vi "LV message server.vi"() -> ()   [LabVIEW 2019, in "mmW_commands.lvlib"]
uses:
  <vilib>/addons/zeromq/socket_type.ctl
  <vilib>/Waveform/WDTOps.llb/WDT Number of Waveform Samples DBL.vi
  mmW_commands.lvlib
  <vilib>/addons/zeromq/zmq_context.lvclass
  <vilib>/addons/zeromq/zmq_socket.lvclass
  <vilib>/addons/zeromq/zeromq.lvlib
  <vilib>/measure/NI_MABase.lvlib
panel:
  out "Config":cluster{"Instrument":string, "Fs":dbl}
  out "size(s)":i32
  out "TX data":waveform(dbl)(graph)
  out "message history":string[](array[string])
  out "error out":errorcluster
  in  "Stop Button":bool
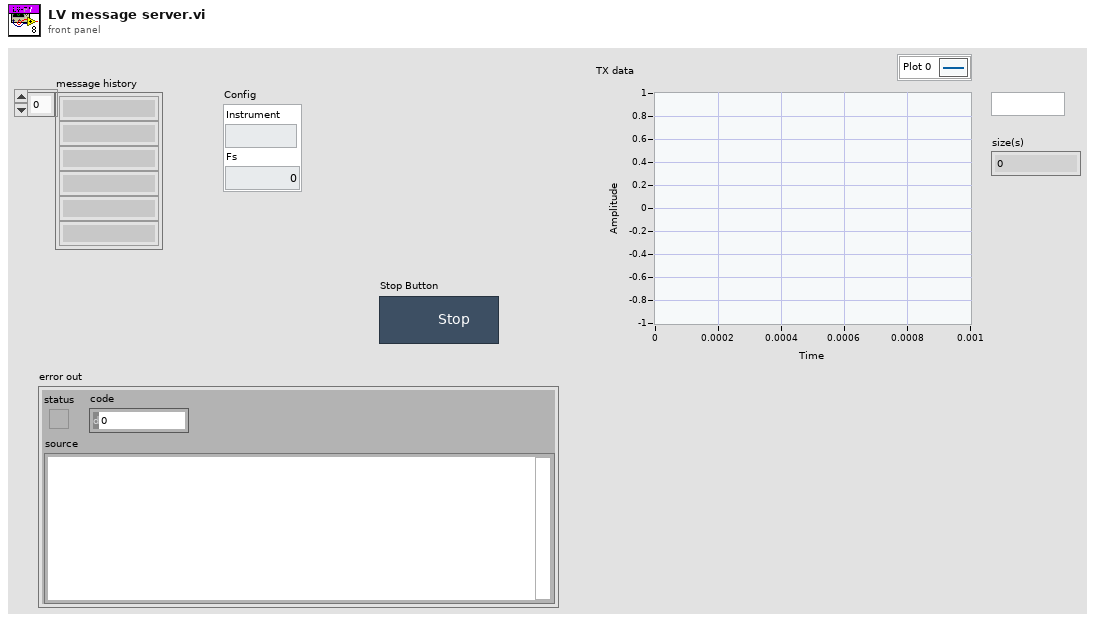
[diagram p1: front panel]
types:
  T1 = typedef "zeromq.lvlib/socket_type.ctl" = enum8{"ZMQ_PAIR", "ZMQ_PUB", "ZMQ_SUB", "ZMQ_REQ", "ZMQ_REP", "ZMQ_DEALER", "ZMQ_ROUTER", "ZMQ_PULL", "ZMQ_PUSH", "ZMQ_XPUB", "ZMQ_XSUB"}
  T2 = enum16{"big-endian, network order", "native, host order", "little-endian"}
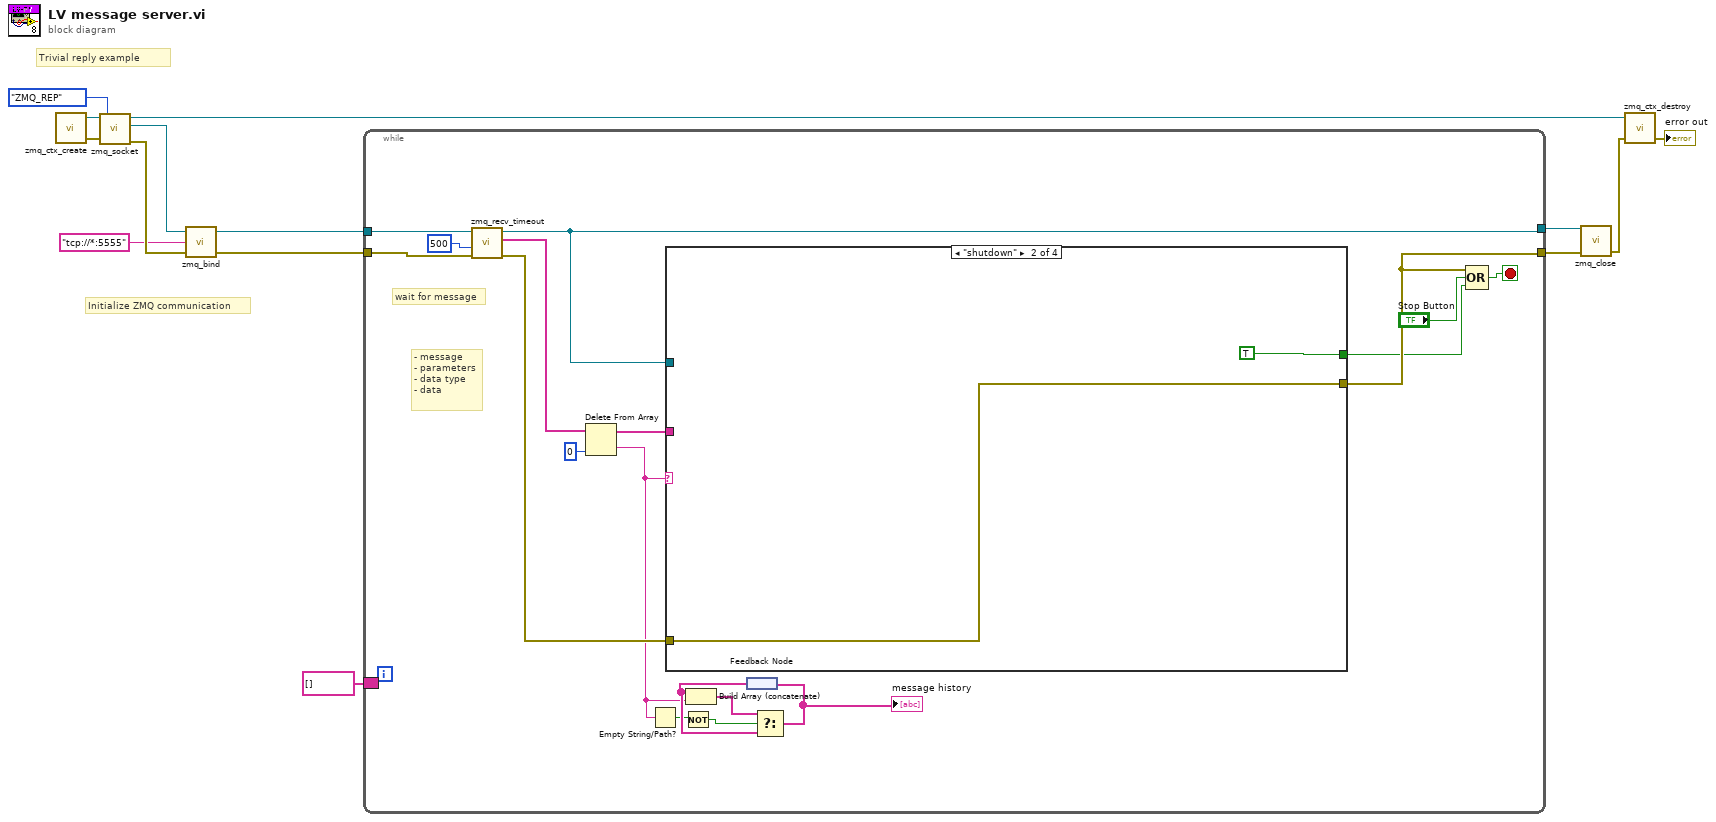
[diagram p0: block diagram]
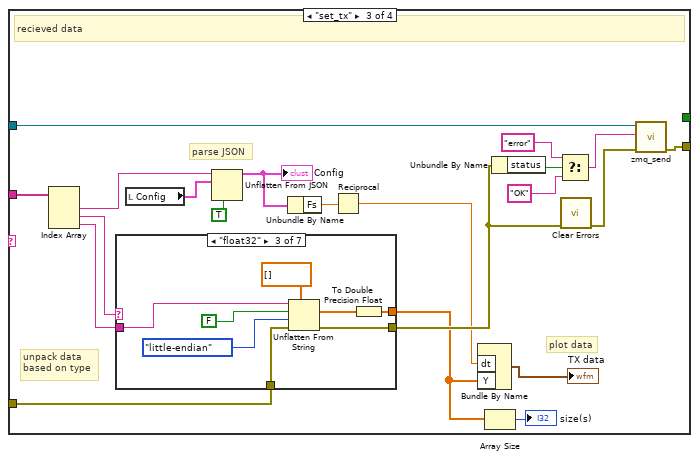
[diagram p3: hidden frame]
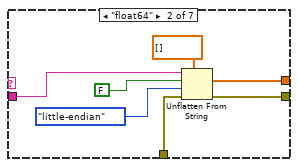
[diagram p5: hidden frame]
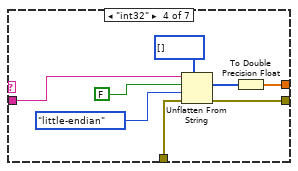
[diagram p6: hidden frame]
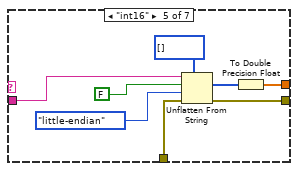
[diagram p7: hidden frame]
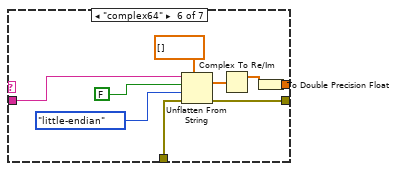
[diagram p8: hidden frame]
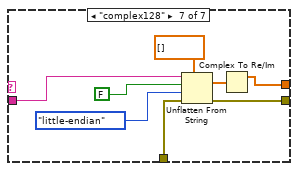
[diagram p9: hidden frame]
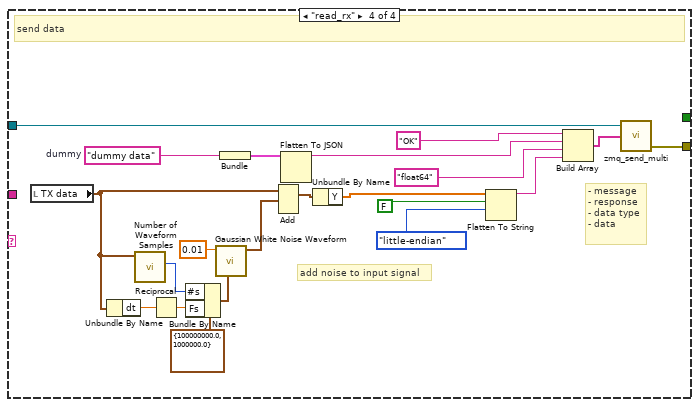
[diagram p10: hidden frame]
diagram:
  # "Initialize ZMQ communication"
  # "Trivial reply example"
  n1 = call <vilib>:"zmq_ctx_create.vi"() -> ("error out"=w12:errorcluster, "context out"=w11:refnum<class "zmq_context.lvclass">)  [unwired: 4 in]
  n2 = call <vilib>:"zmq_socket.vi"("error in"=w12, "socket type"=socket_type."ZMQ_REP", "context in"=w11) -> ("error out"=w14:errorcluster, "socket out"=w13:refnum<class "zmq_socket.lvclass">, "context out"=w5:refnum<class "zmq_context.lvclass">)  [unwired: 2 in]
  n3 = call <vilib>:"zmq_bind.vi"("error in"=w14, "endpoint"="tcp://*:5555", "socket in"=w13) -> ("error out"=w3:errorcluster, "socket out"=w4:refnum<class "zmq_socket.lvclass">)  [unwired: 1 in]
  n4 = while {
    tunnel: w4 -> [w32]
    tunnel: w3 -> [w31]
    tunnel: [w25] -> w8
    tunnel: [w29] -> w7
    border: string[] [] -> [_]
    stop <- w27 stop-if-true
    # "- message\n- parameters\n- data type\n- data"
    # "wait for message"
    n5 = call <vilib>:"zmq_recv_timeout.vi"("error in"=w31, "timeout (ms)"=u32 500, "socket in"=w32) -> ("error out"=w28:errorcluster, "parts"=w20:string[], "socket out"=w29:refnum<class "zmq_socket.lvclass">)  [unwired: 1 in, 1 out]
    n6 = Delete From Array(array=w20, index=0) -> (deleted portion=w17:string, array with subset deleted=w18:string[])  [unwired: 1 in]
    n7 = Empty String/Path?(string/path=w17) -> (empty?=w16:bool)
    n8 = case shown="\"shutdown\"" w17 {
      tunnel: w29 -> [_ _ w51 w124]
      tunnel: w18 -> [_ _ w56 _]
      tunnel: w28 -> [w33 w35 w55 _]
      tunnel: [w33 w35 w41 w115] -> w25
      tunnel: [_ TRUE _ _] -> w24
      frame Default {
      }
      frame "shutdown" {
      }
      frame "set_tx" {
        # "plot data"
        # "unpack data\nbased on type"
        # "parse JSON"
        # "recieved data"
        n9 = Index Array(array=w56) -> (element #1=w44:string, element #2=w52:string, element #3=w53:string)  [unwired: 3 in]
        n10 = case shown="\"float32\"" w52 {
          tunnel: w55 -> [w57 w63 w71 w79 w87 w96 w104]
          tunnel: [w57 w61 w69 w77 w85 w94 w102] -> w50
          tunnel: [_ w60 w65 w73 w81 w89 w98] -> w38
          tunnel: w53 -> [_ w59 w67 w75 w83 w93 w101]
          frame "False", Default {
          }
          frame "float64" {
            n11 = Unflatten From String(type=dbl[] [], binary string=w59, data includes array or string size? (T)=FALSE, byte order (0:big-endian, network order)=T2."little-endian", error in (no error)=w63) -> (value=w60:dbl[], error out=w61:errorcluster)  [unwired: 1 out]
          }
          frame "float32" {
            n12 = Unflatten From String(type=sgl[] [], binary string=w67, data includes array or string size? (T)=FALSE, byte order (0:big-endian, network order)=T2."little-endian", error in (no error)=w71) -> (value=w68:sgl[], error out=w69:errorcluster)  [unwired: 1 out]
            n13 = To Double Precision Float(number=w68) -> (double precision float=w65:dbl[])
          }
          frame "int32" {
            n14 = Unflatten From String(type=i32[] [], binary string=w75, data includes array or string size? (T)=FALSE, byte order (0:big-endian, network order)=T2."little-endian", error in (no error)=w79) -> (value=w76:i32[], error out=w77:errorcluster)  [unwired: 1 out]
            n15 = To Double Precision Float(number=w76) -> (double precision float=w73:dbl[])
          }
          frame "int16" {
            n16 = Unflatten From String(type=i16[] [], binary string=w83, data includes array or string size? (T)=FALSE, byte order (0:big-endian, network order)=T2."little-endian", error in (no error)=w87) -> (value=w84:i16[], error out=w85:errorcluster)  [unwired: 1 out]
            n17 = To Double Precision Float(number=w84) -> (double precision float=w81:dbl[])
          }
          frame "complex64" {
            n18 = Unflatten From String(type=csg[] [], binary string=w93, data includes array or string size? (T)=FALSE, byte order (0:big-endian, network order)=T2."little-endian", error in (no error)=w96) -> (value=w91:csg[], error out=w94:errorcluster)  [unwired: 1 out]
            n19 = Complex To Re/Im(x + iy=w91) -> (x=w90:sgl[])  [unwired: 1 out]
            n20 = To Double Precision Float(number=w90) -> (double precision float=w89:dbl[])
          }
          frame "complex128" {
            n21 = Unflatten From String(type=cdb[] [], binary string=w101, data includes array or string size? (T)=FALSE, byte order (0:big-endian, network order)=T2."little-endian", error in (no error)=w104) -> (value=w99:cdb[], error out=w102:errorcluster)  [unwired: 1 out]
            n22 = Complex To Re/Im(x + iy=w99) -> (x=w98:dbl[])  [unwired: 1 out]
          }
        }
        n23 = local read "Config"() -> (w43:cluster{"Instrument":string, "Fs":dbl})
        n24 = Unflatten From JSON(JSON string=w44, type and defaults=w43, default null elements? (F)=TRUE) -> (value=w40:cluster{"Instrument":string, "Fs":dbl})  [unwired: 4 in, 1 out]
        "Config" <- w40
        n25 = Unbundle By Name(w40) -> ("Fs"=w39:dbl)
        n26 = Reciprocal(x=w39) -> (1/x=w37:dbl)
        n27 = Bundle By Name("dt"=w37, "Y"=w38) -> (→"TX data":waveform(dbl))  [unwired: 1 in]
        n28 = Array Size(array=w38) -> (size(s)=→"size(s)":i32)
        n29 = Unbundle By Name(w50) -> ("status"=w49:bool)
        n30 = Select(t="error" ("data"), s=w49, f="OK" ("data")) -> (s? t:f=w46:string)
        n31 = call <vilib>:"Clear Errors.vi"("error in (no error)"=w50) -> ("error out"=w47:errorcluster)  [unwired: 5 in, 1 out]
        n32 = call <vilib>:"zmq_send.vi"("error in"=w47, "data"=w46, "socket in"=w51) -> ("error out"=w41:errorcluster)  [unwired: 4 in, 1 out]
      }
      frame "read_rx" {
        w120 = "dummy data"  # dummy
        # "add noise to input signal"
        # "- message\n- response\n- data type\n- data"
        # "send data"
        n33 = local read "TX data"() -> (w108:waveform(dbl))
        n34 = Unbundle By Name(w108) -> ("dt"=w106:dbl)
        n35 = call-poly <vilib>:"Number of Waveform Samples.vi"("waveform in"=w108) -> ("number of samples"=w112:i32)  [unwired: 8 in, 2 out]
        n36 = Reciprocal(x=w106) -> (1/x=w107:dbl)
        n37 = Bundle By Name(cluster=cluster{"Fs":dbl, "#s":dbl} {"Fs"=100000000.0, "#s"=1000000.0} ("sampling info"), "#s"=w112, "Fs"=w107) -> (w113:cluster{"Fs":dbl, "#s":dbl})
        n38 = call <vilib>:"Gaussian White Noise Waveform.vi"("sampling info"=w113, "standard deviation"=0.01) -> ("signal out"=w111:waveform(dbl))  [unwired: 8 in, 1 out]
        n39 = Bundle("dummy"=w120) -> (w116:cluster{"dummy":string})  [unwired: 1 in]
        n40 = Add(1:w111, 2:w108) -> (0:w110:waveform(dbl))  [unwired: 1 in, 1 out]
        n41 = Flatten To JSON(anything=w116) -> (JSON string=w117:string)  [unwired: 2 in, 1 out]
        n42 = Unbundle By Name(w110) -> ("Y"=w109:dbl[])
        n43 = Flatten To String(anything=w109, prepend array or string size? (T)=FALSE, byte order (0:big-endian, network order)=T2."little-endian") -> (data string=w118:string)  [unwired: 1 in, 2 out]
        n44 = Build Array("OK" ("element"), w117, "float64" ("element"), w118) -> (w126:string[])
        n45 = call <vilib>:"zmq_send_multi.vi"("parts"=w126, "socket in"=w124) -> ("error out"=w115:errorcluster)  [unwired: 2 in, 1 out]
      }
    }
    n46 = Not(x=w16) -> (.not. x?=w15:bool)
    n47 = feedback #1() -> (w21:string[])
    n48 = Build Array (concatenate)(w21, w17) -> (w23:string[])
    n49 = Select(t=w23, s=w15, f=w21) -> (s? t:f=w22:string[])
    "message history" <- w22
    n50 = feedback-in #1(w22) -> ()
    n51 = Compound Arithmetic op=OR(w25, "Stop Button", w24) -> (w27:bool)
  }
  n52 = call <vilib>:"zmq_close.vi"("error in"=w8, "socket"=w7) -> ("error out"=w6:errorcluster)  [unwired: 3 in]
  n53 = call <vilib>:"zmq_ctx_destroy.vi"("error in"=w6, "context in"=w5) -> ("error out"=→"error out":errorcluster)  [unwired: 3 in]
